vi "Main.vi"() -> ()   [LabVIEW 2015]
doc: "The myRIO Project template acquires acceleration data from the onboard accelerometer and displays the changes of acceleration values in a waveform chart."
uses:
  <vilib>/myRIO/Instrument Drivers/Onboard IO/PWM/typedefs/PWM Reference.ctl
  <vilib>/myRIO/Common/Instrument Driver Framework/Utilities/typedefs/myRIO Generic Hardware Reference.ctl
  <vilib>/myRIO/Common/Instrument Driver Framework/Utilities/typedefs/Hardware Version Enum.ctl
  <vilib>/myRIO/Common/Instrument Driver Framework/Utilities/typedefs/myRIO v1.0 Reference.ctl
  <vilib>/myRIO/Common/Instrument Driver Framework/Utilities/typedefs/Generic FPGA Reference.ctl
  <vilib>/myRIO/Common/Instrument Driver Framework/myRIO v1.0/PWM/typedefs/PWM Channels Enum.ctl
  <vilib>/myRIO/Instrument Drivers/Onboard IO/PWM/typedefs/PWM Configuration.ctl
  <vilib>/userdefined/High Color/nirio_resource_hc.ctl
  <vilib>/myRIO/Instrument Drivers/Onboard IO/AI/typedefs/AI Reference.ctl
  <vilib>/myRIO/Common/Instrument Driver Framework/myRIO v1.0/AI/typedefs/AI Channels List.ctl
  <vilib>/myRIO/Common/Instrument Driver Framework/myRIO v1.0/AI/typedefs/AI Channels Enum.ctl
  <vilib>/myRIO/Common/Instrument Driver Framework/Utilities/typedefs/Analog Scaling Constants List.ctl
  <vilib>/myRIO/Common/Instrument Driver Framework/Utilities/typedefs/Analog Scaling Constants.ctl
  <vilib>/myRIO/Instrument Drivers/Onboard IO/DIO/typedefs/DIO Reference.ctl
  <vilib>/myRIO/Common/Instrument Driver Framework/myRIO v1.0/DIO/typedefs/DIO Channels List.ctl
  <vilib>/myRIO/Common/Instrument Driver Framework/myRIO v1.0/DIO/typedefs/DIO Channels Enum.ctl
  <vilib>/myRIO/Instrument Drivers/Onboard Devices/Accelerometer/typedefs/Accelerometer Reference.ctl
  <vilib>/myRIO/Common/Instrument Driver Framework/myRIO v1.0/Accelerometer/typedefs/Accelerometer Channels List.ctl
  <vilib>/myRIO/Common/Instrument Driver Framework/myRIO v1.0/Accelerometer/typedefs/Accelerometer Channels Enum.ctl
  <vilib>/myRIO/Common/Instrument Driver Framework/Utilities/vis/Is FPGA Ref Available.vi
  <vilib>/myRIO/Common/Instrument Driver Framework/myRIO v1.0/DIO/vis/myRIO v1.1 Open DIO.vi
  <vilib>/myRIO/Instrument Drivers/Onboard IO/DIO/vis/Write.vi
  <vilib>/myRIO/Instrument Drivers/Onboard IO/DIO/vis/Read.vi
  <vilib>/myRIO/Common/Instrument Driver Framework/myRIO v1.0/PWM/vis/myRIO v1.1 Open PWM.vi
  <vilib>/myRIO/Instrument Drivers/Onboard IO/PWM/vis/Set Duty Cycle and Frequency.vi
  <vilib>/myRIO/Common/Instrument Driver Framework/myRIO v1.0/AI/vis/myRIO v1.1 Open AI.vi
  <vilib>/myRIO/Instrument Drivers/Onboard IO/AI/vis/Read.vi
  <vilib>/myRIO/Common/Instrument Driver Framework/myRIO v1.0/Accelerometer/vis/myRIO v1.1 Open Accelerometer.vi
  <vilib>/myRIO/Instrument Drivers/Onboard Devices/Accelerometer/vis/Read.vi
  <vilib>/myRIO/Common/Instrument Driver Framework/Utilities/vis/Validate Channels.vi
  <vilib>/myRIO/Common/Instrument Driver Framework/myRIO v1.0/DIO/vis/myRIO v1.0 Reserve DIO.vi
  <vilib>/myRIO/Common/Instrument Driver Framework/myRIO v1.0/PWM/vis/myRIO v1.0 Reserve PWM.vi
  <vilib>/myRIO/Common/Instrument Driver Framework/myRIO v1.0/AI/vis/myRIO v1.0 Reserve AI.vi
  <vilib>/myRIO/Common/Instrument Driver Framework/myRIO v1.0/Accelerometer/vis/myRIO v1.0 Reserve Accelerometer.vi
  <vilib>/myRIO/Common/Instrument Driver Framework/myRIO v1.0/UART/vis/myRIO v1.0 Close UART.vi
  <vilib>/myRIO/Common/Instrument Driver Framework/myRIO v1.0/Resource Manager/vis/myRIO v1.0 Reserve Channel List.vi
  <vilib>/myRIO/Common/Instrument Driver Framework/myRIO v1.0/DIO/vis/myRIO v1.0 Build MUX Configuration DIO.vi
  <vilib>/myRIO/Common/Instrument Driver Framework/myRIO v1.0/PWM/vis/myRIO v1.0 Build MUX Configuration PWM.vi
  <vilib>/myRIO/Common/Instrument Driver Framework/myRIO v1.0/AI/vis/myRIO v1.0 Build MUX Configuration AI.vi
  <vilib>/myRIO/Common/Instrument Driver Framework/myRIO v1.0/Accelerometer/vis/myRIO v1.0 Build MUX Configuration Accelerometer.vi
  <vilib>/myRIO/Common/Instrument Driver Framework/myRIO v1.0/Resource Manager/vis/myRIO v1.0 Reserve Channel.vi
  <vilib>/myRIO/Common/Instrument Driver Framework/myRIO v1.0/Resource Manager/vis/myRIO v1.0 Unreserve Channel.vi
  <vilib>/myRIO/Common/Instrument Driver Framework/myRIO v1.0/Resource Manager/vis/myRIO v1.0 Create Configuration List.vi
  <vilib>/myRIO/Common/Instrument Driver Framework/myRIO v1.0/Resource Manager/vis/myRIO v1.0 Build Mutex Name.vi
  <vilib>/Utility/VariantDataType/GetNumericInfo.vi
  <vilib>/Utility/error.llb/Error Cluster From Error Code.vi
  <vilib>/myRIO/Common/Instrument Driver Framework/myRIO v1.0/myRIO v1.1 Open.vi
  <vilib>/myRIO/Common/Instrument Driver Framework/Utilities/vis/IO Manager.vi
  <vilib>/myRIO/Common/Instrument Driver Framework/Utilities/vis/Configuration Manager.vi
  <vilib>/myRIO/Common/Instrument Driver Framework/myRIO v1.0/Resource Manager/vis/myRIO v1.0 Configure IO.vi
  <vilib>/myRIO/Common/Instrument Driver Framework/myRIO v1.0/myRIO v1.0 Close.vi
  <vilib>/myRIO/Common/Instrument Driver Framework/myRIO v1.0/PWM/vis/myRIO v1.0 Write PWM.vi
  <vilib>/myRIO/Common/Instrument Driver Framework/myRIO v1.0/AI/vis/myRIO v1.0 Get Scaling Constants AI.vi
  <vilib>/myRIO/Common/Instrument Driver Framework/myRIO v1.0/AI/vis/myRIO v1.0 Read AI.vi
  <vilib>/addons/control/pid/pid.llb/PID (DBL).vi
  <vilib>/myRIO/Common/Instrument Driver Framework/myRIO v1.0/DIO/vis/myRIO v1.0 Read DIO.vi
  <vilib>/myRIO/Common/Instrument Driver Framework/myRIO v1.0/DIO/vis/myRIO v1.0 Write DIO.vi
  <vilib>/myRIO/Common/Instrument Driver Framework/myRIO v1.0/Accelerometer/vis/myRIO v1.0 Get Scaling Constant Accelerometer.vi
  <vilib>/myRIO/Common/Instrument Driver Framework/myRIO v1.0/Accelerometer/vis/myRIO v1.0 Read Accelerometer.vi
  <vilib>/myRIO/Common/Instrument Driver Framework/Utilities/vis/FPGA Ref Manager.vi
  <vilib>/myRIO/Common/Instrument Driver Framework/myRIO v1.0/myRIO v1.0 Reset FPGA.vi
  <vilib>/myRIO/Common/Instrument Driver Framework/myRIO v1.0/IRQ/vis/myRIO v1.0 IRQ Info FGV.vi
  <vilib>/myRIO/Common/Instrument Driver Framework/myRIO v1.0/IRQ/vis/myRIO v1.0 Timer IRQ Info FGV.vi
  <vilib>/myRIO/Common/Instrument Driver Framework/myRIO v1.0/IRQ/vis/myRIO v1.0 ISR Agent.vi
  <vilib>/myRIO/Express VI/Onboard IO/PWM/PWM Express VI.xnode
  <vilib>/myRIO/Instrument Drivers/Onboard IO/PWM/vis/myRIO PWM Open.xnode
  <vilib>/myRIO/Express VI/Onboard IO/AI/AI Express VI.xnode
  <vilib>/myRIO/Instrument Drivers/Onboard IO/AI/vis/myRIO AI Open.xnode
  <vilib>/myRIO/Express VI/Onboard IO/DI/DI Express VI.xnode
  <vilib>/myRIO/Instrument Drivers/Onboard IO/DIO/vis/myRIO DIO Open.xnode
  <vilib>/myRIO/Express VI/Onboard IO/DO/DO Express VI.xnode
  <vilib>/myRIO/Express VI/Onboard Devices/Accelerometer/Accelerometer Express VI.xnode
  <vilib>/myRIO/Instrument Drivers/Onboard Devices/Accelerometer/vis/myRIO Accelerometer Open.xnode
  <vilib>/myRIO/Instrument Drivers/Utilities/Utilities.lvlib
  <vilib>/myRIO/Instrument Drivers/Onboard Devices/Accelerometer/Accelerometer.lvlib
  <vilib>/myRIO/Instrument Drivers/Onboard IO/PWM/PWM.lvlib
  <vilib>/myRIO/Instrument Drivers/Onboard IO/DIO/DIO.lvlib
  <vilib>/myRIO/Instrument Drivers/Onboard IO/AI/AI.lvlib
  <vilib>/addons/control/pid/NI_PID_pid.lvlib
panel:
  in  "turn":bool
  out "波形图表 2":dbl(graph)
  out "波形图表":dbl(graph)
  out "数值 3":dbl
  out "数值 2":dbl
  out "数值":dbl
  in  "PID gains":T1={"proportional gain (Kc)"=1.0, "integral time (Ti, min)"=0.01, "derivative time (Td, min)"=0.0} caption="PID增益" {"derivative time (Td, min)" format="%.3f"; "integral time (Ti, min)" format="%.3f"; "proportional gain (Kc)" format="%.3f"}
  out "Acceleration":T2(graph)
  out "error out":errorcluster
  in  "Stop":bool
  # "Overview: The myRIO Project template acquires acceleration data from the onboard accelerometer and displays the changes of acceleration values in a waveform chart.\nInstructions:\n1. Check the myRIO target IP address in the project and make sure the target IP address is correct. \n2. Run this VI."
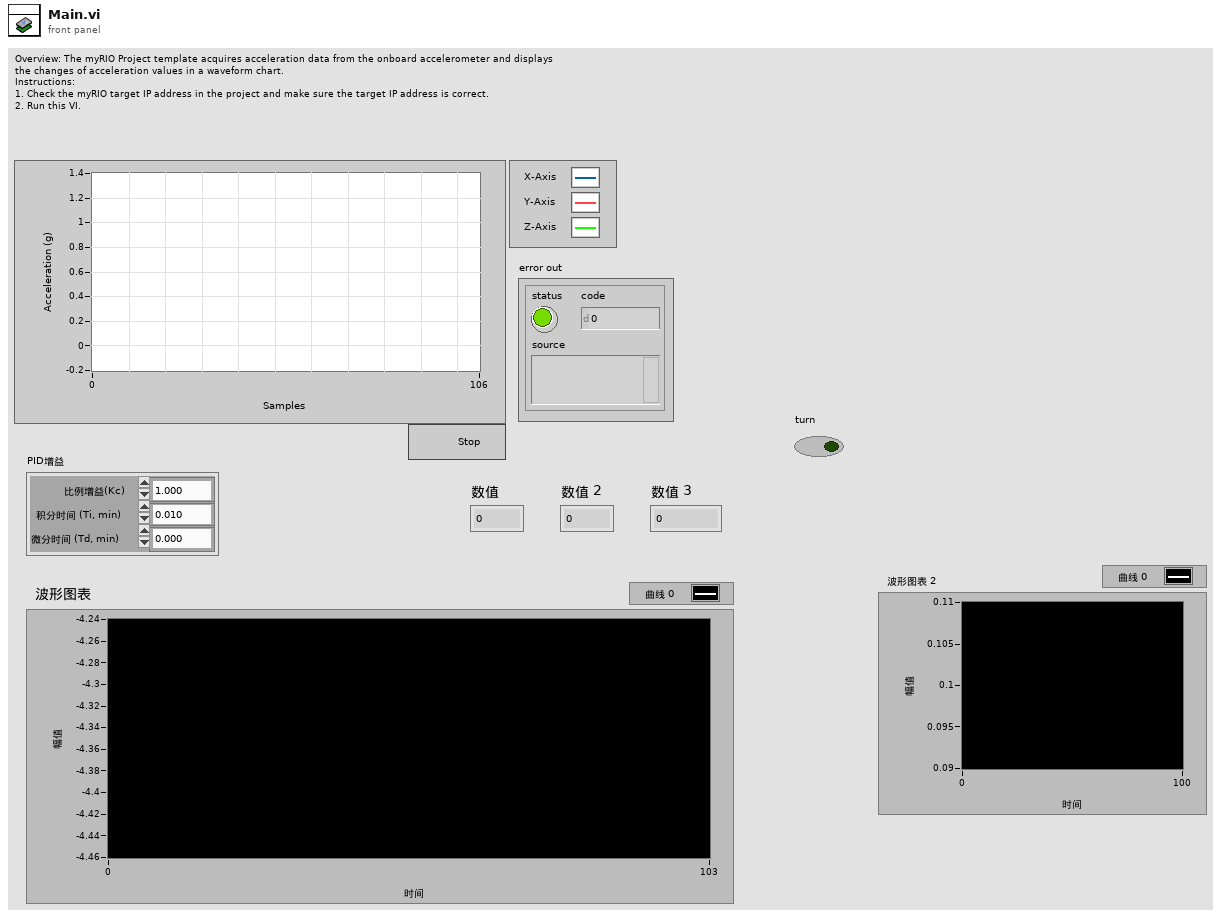
[diagram p1: front panel]
types:
  T1 = cluster{"proportional gain (Kc)":dbl, "integral time (Ti, min)":dbl, "derivative time (Td, min)":dbl}
  T2 = cluster{"X-Axis":dbl, "Y-Axis":dbl, "Z-Axis":dbl}
  T3 = typedef "PWM.lvlib/PWM Reference.ctl" = cluster{"myRIO Reference":T4, "PWM Channels Enum":T8, "PWM Configuration":T9}
  T4 = typedef "myRIO Generic Hardware Reference.ctl" = cluster{"myRIO Model":T5, "myRIO Hardware Reference":T6}
  T5 = typedef "Hardware Version Enum.ctl" = enum16{"Unknown", "myRIO-1900", "myRIO-1950", "roboRIO"}
  T6 = typedef "myRIO v1.0 Reference.ctl" = cluster{"Generic FPGA Reference":T7, "Allow multiple opens":bool}
  T7 = typedef "Generic FPGA Reference.ctl" = refnum<k20>
  T8 = typedef "PWM Channels Enum.ctl" = enum16{"Not Connected", "C/PWM0", "C/PWM1", "A/PWM0", "A/PWM1", "A/PWM2", "B/PWM0", "B/PWM1", "B/PWM2", "PWM/PWM0", "PWM/PWM1", "PWM/PWM2", "PWM/PWM3", "PWM/PWM4", "PWM/PWM5", "PWM/PWM6", "PWM/PWM7", "PWM/PWM8", "PWM/PWM9"}
  T9 = typedef "PWM.lvlib/PWM Configuration.ctl" = cluster{"Frequency":dbl, "Duty Cycle":dbl}
  T10 = typedef "nirio_resource_hc.ctl" = tag
  T11 = typedef "DIO.lvlib/DIO Reference.ctl" = cluster{"myRIO Reference":T4, "DIO Channels List":T12}
  T12 = typedef "DIO Channels List.ctl" = T13[]
  T13 = typedef "DIO Channels Enum.ctl" = enum16{"Not Connected", "C/DIO0", "C/DIO1", "C/DIO2", "C/DIO3", "C/DIO4", "C/DIO5", "C/DIO6", "C/DIO7", "A/DIO0", "A/DIO1", "A/DIO2", "A/DIO3", "A/DIO4", "A/DIO5", "A/DIO6", "A/DIO7", "A/DIO8", "A/DIO9", "A/DIO10", "A/DIO11", "A/DIO12", "A/DIO13", "A/DIO14", "A/DIO15", "B/DIO0", "B/DIO1", "B/DIO2", "B/DIO3", "B/DIO4", "B/DIO5", "B/DIO6", "B/DIO7", "B/DIO8", "B/DIO9", "B/DIO10", "B/DIO11", "B/DIO12", "B/DIO13", "B/DIO14", "B/DIO15", "LED0", "LED1", "LED2", "LED3", "Button0", "DIO/DIO0", "DIO/DIO1", "DIO/DIO2", "DIO/DIO3", "DIO/DIO4", "DIO/DIO5", "DIO/DIO6", "DIO/DIO7", "DIO/DIO8", "DIO/DIO9", "SPI/CS0", "SPI/CS1", "SPI/CS2", "SPI/CS3", "LED RADIO (Green)", "LED RADIO (Red)", "LED COMM (Green)", "LED COMM (Red)", "LED MODE (Green)", "LED MODE (Red)"}
  T14 = typedef "AI.lvlib/AI Reference.ctl" = cluster{"myRIO Reference":T4, "AI Channels List":T15, "AI Scaling Constants List":T17}
  T15 = typedef "AI Channels List.ctl" = T16[]
  T16 = typedef "AI Channels Enum.ctl" = enum16{"Not Connected", "AudioIn/Left", "AudioIn/Right", "C/AI0", "C/AI1", "A/AI0", "A/AI1", "A/AI2", "A/AI3", "B/AI0", "B/AI1", "B/AI2", "B/AI3", "AI/AI0", "AI/AI1", "AI/AI2", "AI/AI3"}
  T17 = typedef "Analog Scaling Constants List.ctl" = T18[]
  T18 = typedef "Analog Scaling Constants.ctl" = cluster{"LSB Weight (Volts)":dbl, "Offset (Volts)":dbl, "Signed?":bool}
  T19 = typedef "Accelerometer.lvlib/Accelerometer Reference.ctl" = cluster{"myRIO Reference":T4, "Accelerometer Channels List":T20, "LSB Weight":dbl}
  T20 = typedef "Accelerometer Channels List.ctl" = T21[]
  T21 = typedef "Accelerometer Channels Enum.ctl" = enum16{"Not Connected", "X-Axis", "Y-Axis", "Z-Axis"}
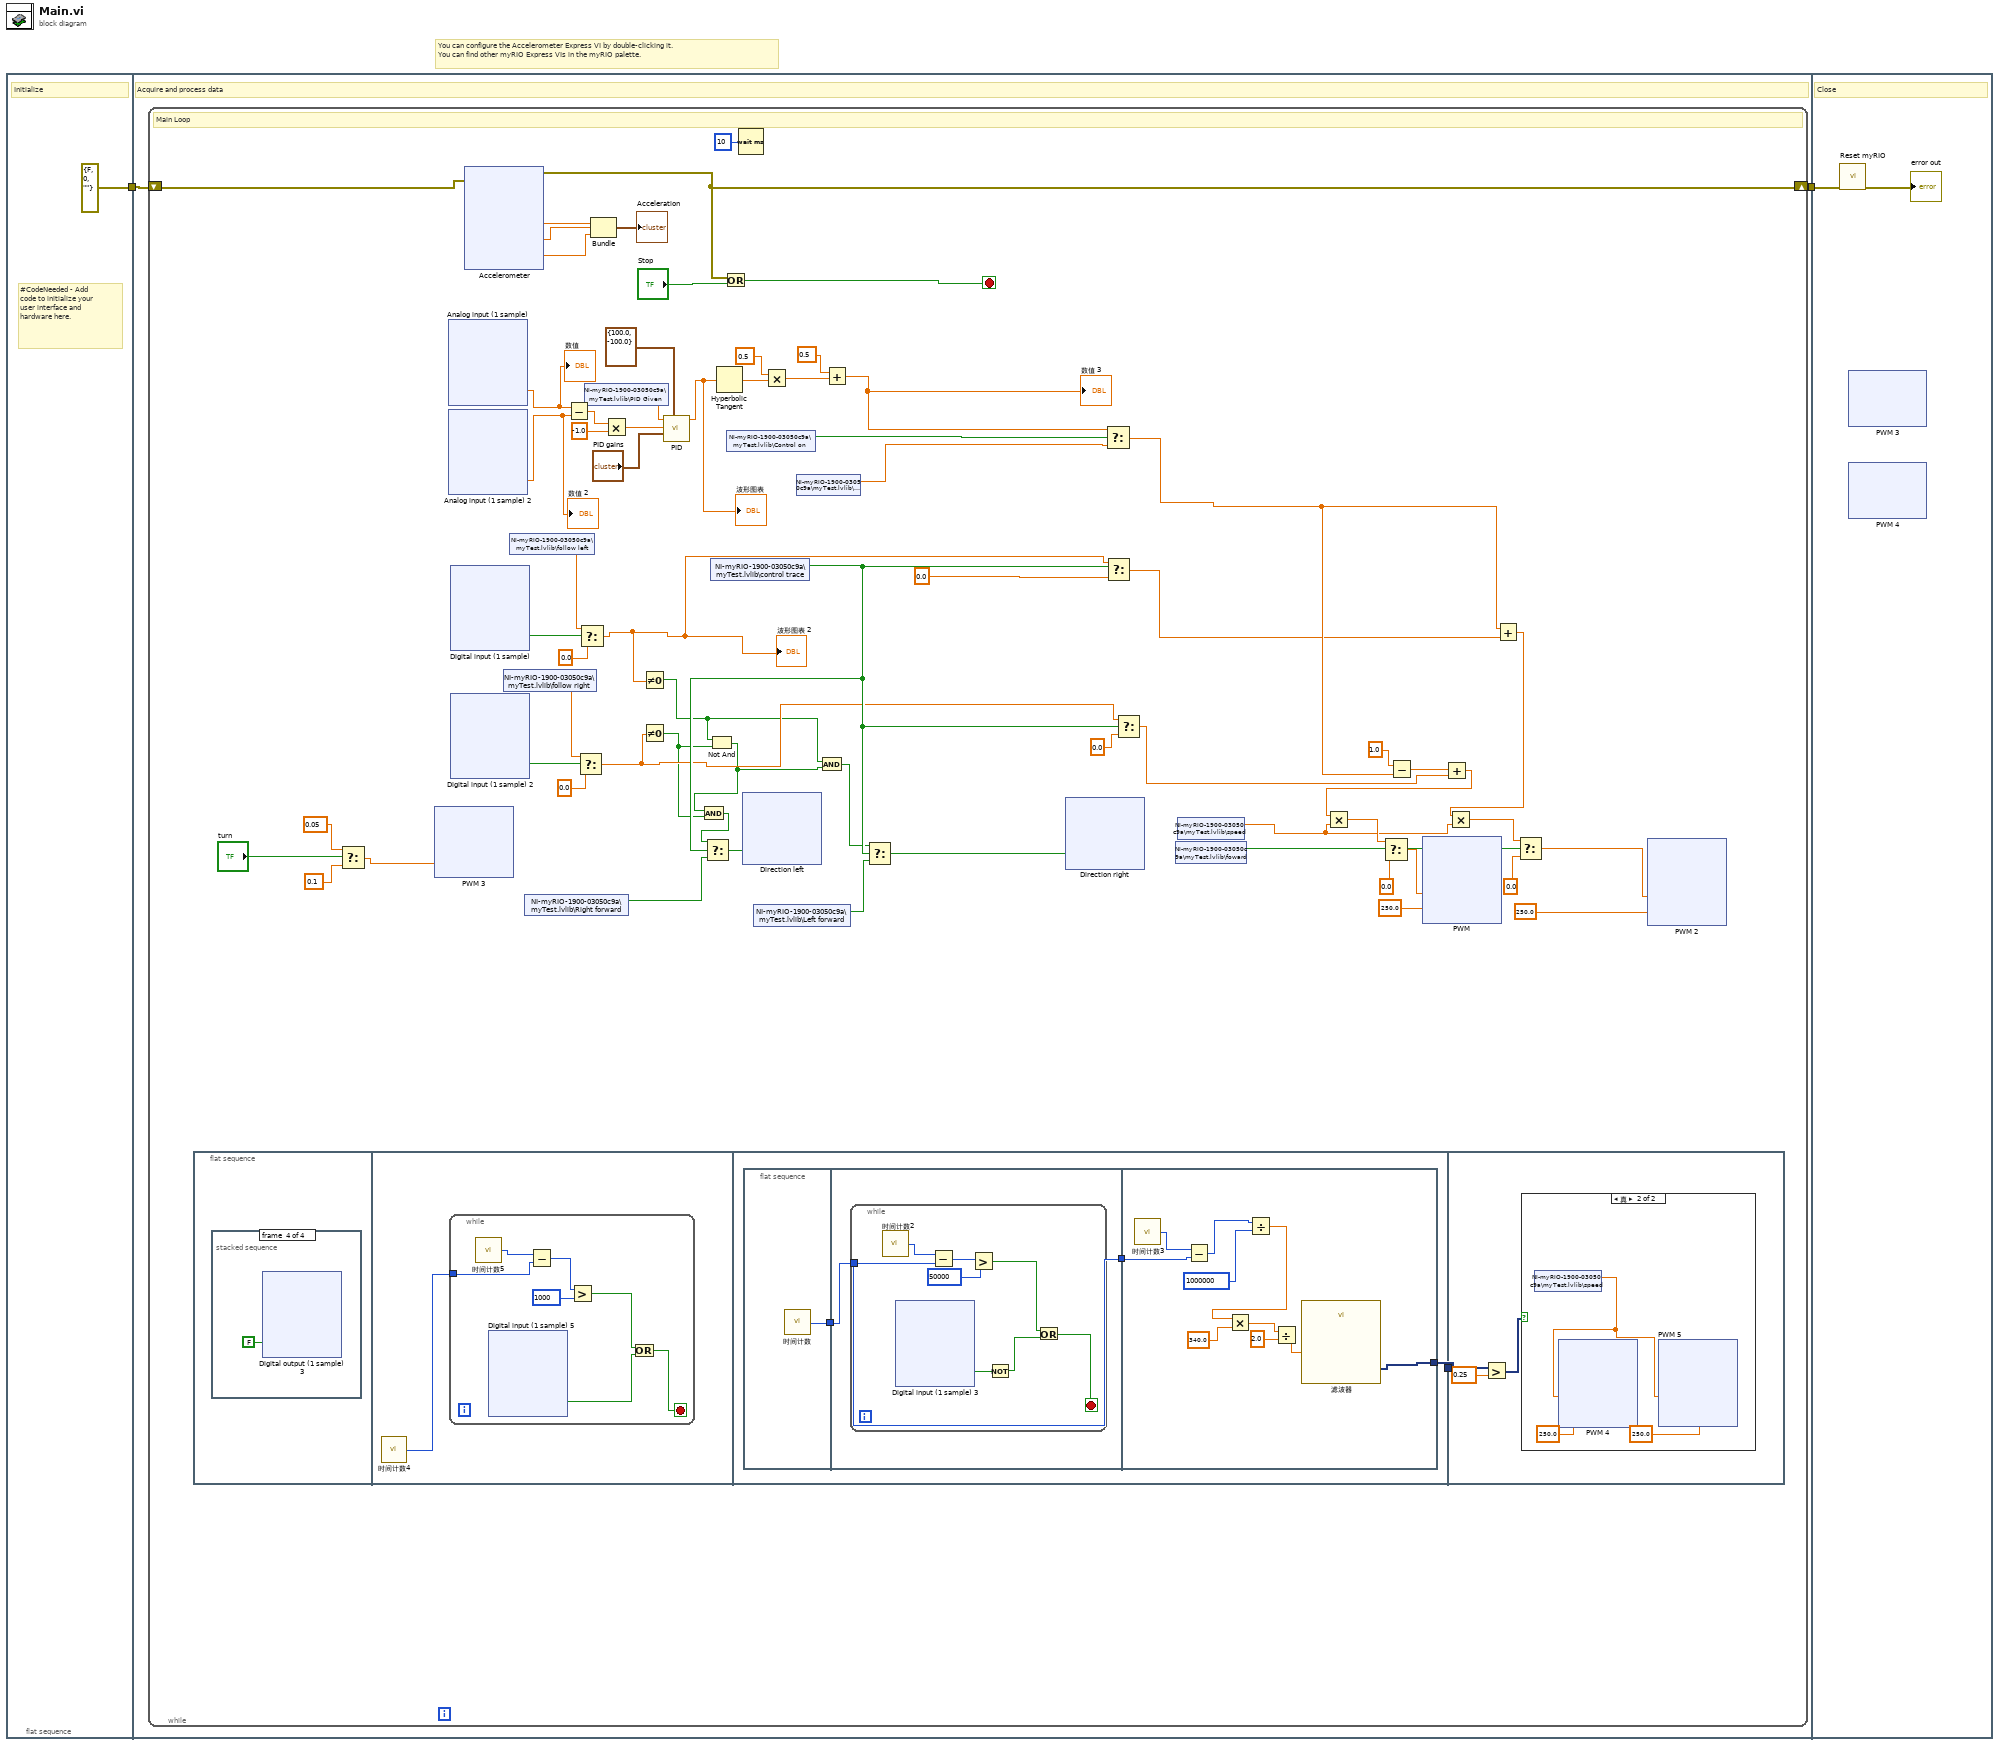
[diagram p0: block diagram]
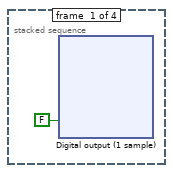
[diagram p2: hidden frame]
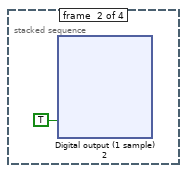
[diagram p3: hidden frame]
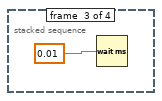
[diagram p4: hidden frame]
diagram:
  # "You can configure the Accelerometer Express VI by double-clicking it.\nYou can find other myRIO Express VIs in the myRIO palette."
  n1 = flat-sequence {
    tunnel: [errorcluster {"status"=FALSE, "code"=0, "source"=""} ("error in (no error)")] -> w2
    tunnel: w2 -> [w5]
    tunnel: [w4] -> w1
    tunnel: w1 -> [w718]
    frame #0 {
      # "#CodeNeeded - Add code to initialize your user interface and hardware here."
      # "Initialize"
    }
    frame #1 {
      # "Acquire and process data"
      n2 = while {
        shift-right: [w68] -> w4
        shift-left: w5 -> [w64]
        stop <- w71 stop-if-true
        # "Main Loop"
        n3 = flat-sequence {
          tunnel: [w260] -> w6
          tunnel: w6 -> [w320]
          frame #0 {
            n4 = stacked-sequence {
              frame #0 {
                n5 = xnode "Digital output (1 sample)"("A/DIO10 (Pin 31)"=FALSE) -> ()  [unwired: 1 in, 1 out]
              }
              frame #1 {
                n6 = xnode "Digital output (1 sample) 2"("A/DIO10 (Pin 31)"=TRUE) -> ()  [unwired: 1 in, 1 out]
              }
              frame #2 {
                n7 = Wait (ms)(milliseconds to wait=0.01 ("等待时间（毫秒）")) -> ()  [unwired: 1 out]
              }
              frame #3 {
                n8 = xnode "Digital output (1 sample) 3"("A/DIO10 (Pin 31)"=FALSE) -> ()  [unwired: 1 in, 1 out]
              }
            }
          }
          frame #1 {
            n9 = call "时间计数4"() -> ("Tick Count(uSec)"=w217:u32)
            n10 = while {
              tunnel: w217 -> [w223]
              stop <- w218 stop-if-true
              n11 = call "时间计数5"() -> ("Tick Count(uSec)"=w224:u32)
              n12 = xnode "Digital input (1 sample) 5"() -> ("A/DIO7 (Pin 25)"=w220:bool)  [unwired: 1 in, 1 out]
              n13 = Subtract(x=w224, y=w223) -> (x-y=w222:u32)
              n14 = Greater?(x=w222, y=u32 1000) -> (0:w219:bool)
              n15 = Or(x=w219, y=w220) -> (x .or. y?=w218:bool)
            }
          }
          frame #2 {
            n16 = flat-sequence {
              tunnel: [w263] -> w262
              tunnel: w262 -> [w264]
              tunnel: [w264] -> w261
              tunnel: w261 -> [w316]
              tunnel: [w308] -> w260
              frame #0 {
                n17 = call "时间计数"() -> ("Tick Count(uSec)"=w263:u32)
              }
              frame #1 {
                n18 = while {
                  tunnel: w264 -> [w271]
                  stop <- w265 stop-if-true
                  n19 = call "时间计数2"() -> ("Tick Count(uSec)"=w272:u32)
                  n20 = xnode "Digital input (1 sample) 3"() -> ("A/DIO7 (Pin 25)"=w268:bool)  [unwired: 1 in, 1 out]
                  n21 = Subtract(x=w272, y=w271) -> (x-y=w270:u32)
                  n22 = Greater?(x=w270, y=u32 50000) -> (0:w267:bool)
                  n23 = Not(x=w268) -> (.not. x?=w266:bool)
                  n24 = Or(x=w267, y=w266) -> (x .or. y?=w265:bool)
                }
              }
              frame #2 {
                n25 = call "时间计数3"() -> ("Tick Count(uSec)"=w317:u32)
                n26 = Subtract(x=w317, y=w316) -> (x-y=w315:u32)
                n27 = Divide(x=w315, y=u32 1000000) -> (x/y=w311:dbl)
                n28 = Multiply(x=w311, y=340.0) -> (x*y=w312:dbl)
                n29 = Divide(x=w312, y=2.0) -> (x/y=w309:dbl)
                n30 = call "滤波器"("Signal"=w309) -> ("Filtered Signal"=w308:dynamicdata)  [unwired: 9 in, 1 out]
              }
            }
          }
          frame #3 {
            n31 = Greater?(x=w320, y=0.25) -> (0:w318:dynamicdata)
            n32 = case shown="真" w318 {
              frame False {
              }
              frame True {
                n33 = shared-variable "NI-myRIO-1900-03050c9a\\myTest.lvlib\\speed"() -> (w321:dbl)  [unwired: 1 in, 1 out]
                n34 = xnode "PWM 4"("Duty Cycle"=w321, "Frequency [Hz]"=250.0) -> ()  [unwired: 1 in, 1 out]
                n35 = xnode "PWM 5"("Duty Cycle"=w321, "Frequency [Hz]"=250.0) -> ()  [unwired: 1 in, 1 out]
              }
            }
          }
        }
        n36 = Select(t=0.05, s="turn", f=0.1) -> (s? t:f=w10:dbl)
        n37 = xnode "PWM 3"("Duty Cycle"=w10) -> ()  [unwired: 1 in, 1 out]
        n38 = xnode "Analog input (1 sample)"() -> ("A/AI2 (Pin 7)"=w47:dbl)  [unwired: 1 in, 1 out]
        "数值" <- w47
        n39 = xnode "Analog input (1 sample) 2"() -> ("A/AI1 (Pin 5)"=w48:dbl)  [unwired: 1 in, 1 out]
        "数值 2" <- w48
        n40 = xnode "Digital input (1 sample)"() -> ("A/DIO1 (Pin 13)"=w27:bool)  [unwired: 1 in, 1 out]
        n41 = xnode "Digital input (1 sample) 2"() -> ("A/DIO0 (Pin 11)"=w28:bool)  [unwired: 1 in, 1 out]
        n42 = xnode "Accelerometer"("error in (no error)"=w64) -> ("X-Axis"=w66:dbl, "Y-Axis"=w65:dbl, "Z-Axis"=w67:dbl, "error out"=w68:errorcluster)
        n43 = shared-variable "NI-myRIO-1900-03050c9a\\myTest.lvlib\\follow right"() -> (w23:dbl)  [unwired: 1 in, 1 out]
        n44 = shared-variable "NI-myRIO-1900-03050c9a\\myTest.lvlib\\follow left"() -> (w24:dbl)  [unwired: 1 in, 1 out]
        n45 = shared-variable "NI-myRIO-1900-03050c9a\\myTest.lvlib\\Right forward"() -> (w22:bool)  [unwired: 1 in, 1 out]
        n46 = Subtract(x=w47, y=w48) -> (x-y=w40:dbl)
        n47 = Select(t=w23, s=w28, f=0.0 ("x")) -> (s? t:f=w17:dbl)
        n48 = Select(t=w24, s=w27, f=0.0 ("x")) -> (s? t:f=w16:dbl)
        "波形图表 2" <- w16
        n49 = shared-variable "NI-myRIO-1900-03050c9a\\myTest.lvlib\\PID Given"() -> (w41:dbl)  [unwired: 1 in, 1 out]
        n50 = Bundle("X-Axis"=w66, "Y-Axis"=w65, "Z-Axis"=w67) -> (→"Acceleration":T2)  [unwired: 1 in]
        n51 = Multiply(x=w40, y=-1.0) -> (x*y=w38:dbl)
        n52 = Not Equal To 0?(x=w16) -> (x != 0?=w13:bool)
        n53 = Not Equal To 0?(x=w17) -> (x != 0?=w15:bool)
        n54 = call-poly <vilib>:"PID.vi"("output range"=cluster{"output high":dbl, "output low":dbl} {"output high"=100.0, "output low"=-100.0}, "PID gains"="PID gains", "process variable"=w38, "setpoint"=w41) -> ("output"=w42:dbl)  [unwired: 6 in, 1 out]
        "波形图表" <- w42
        n55 = Not And(1:w15, 2:w13) -> (0:w12:bool)
        n56 = And(x=w12, y=w15) -> (x .and. y?=w14:bool)
        n57 = shared-variable "NI-myRIO-1900-03050c9a\\myTest.lvlib\\control trace"() -> (w18:bool)  [unwired: 1 in, 1 out]
        n58 = Select(t=w14, s=w18, f=w22) -> (s? t:f=w21:bool)
        n59 = Hyperbolic Tangent(1:w42) -> (0:w45:dbl)
        n60 = Or(x=w68, y="Stop") -> (x .or. y?=w71:bool)
        n61 = shared-variable "NI-myRIO-1900-03050c9a\\myTest.lvlib\\Control on"() -> (w50:bool)  [unwired: 1 in, 1 out]
        n62 = Wait (ms)(milliseconds to wait=u32 10) -> ()  [unwired: 1 out]
        n63 = xnode "Direction left"("B/DIO3 (Pin 17)"=w21) -> ()  [unwired: 1 in, 1 out]
        n64 = shared-variable "NI-myRIO-1900-03050c9a\\myTest.lvlib\\Left forward"() -> (w19:bool)  [unwired: 1 in, 1 out]
        n65 = Multiply(x=0.5, y=w45) -> (x*y=w43:dbl)
        n66 = shared-variable "NI-myRIO-1900-03050c9a\\myTest.lvlib\\angle"() -> (w49:dbl)  [unwired: 1 in, 1 out]
        n67 = And(x=w13, y=w12) -> (x .and. y?=w11:bool)
        n68 = Add(x=0.5, y=w43) -> (x+y=w46:dbl)
        "数值 3" <- w46
        n69 = Select(t=w11, s=w18, f=w19) -> (s? t:f=w20:bool)
        n70 = xnode "Direction right"("A/DIO3 (Pin 17)"=w20) -> ()  [unwired: 1 in, 1 out]
        n71 = Select(t=w46, s=w50, f=w49) -> (s? t:f=w31:dbl)
        n72 = Select(t=w16, s=w18, f=0.0) -> (s? t:f=w30:dbl)
        n73 = Select(t=w17, s=w18, f=0.0) -> (s? t:f=w29:dbl)
        n74 = shared-variable "NI-myRIO-1900-03050c9a\\myTest.lvlib\\foward"() -> (w57:bool)  [unwired: 1 in, 1 out]
        n75 = shared-variable "NI-myRIO-1900-03050c9a\\myTest.lvlib\\speed"() -> (w37:dbl)  [unwired: 1 in, 1 out]
        n76 = Subtract(x=1.0, y=w31) -> (x-y=w33:dbl)
        n77 = Add(x=w33, y=w29) -> (x+y=w32:dbl)
        n78 = Multiply(x=w32, y=w37) -> (x*y=w55:dbl)
        n79 = Select(t=w55, s=w57, f=0.0) -> (s? t:f=w58:dbl)
        n80 = xnode "PWM"("Duty Cycle"=w58, "Frequency [Hz]"=250.0) -> ()  [unwired: 1 in, 1 out]
        n81 = Add(x=w31, y=w30) -> (x+y=w34:dbl)
        n82 = Multiply(x=w34, y=w37) -> (x*y=w54:dbl)
        n83 = Select(t=w54, s=w57, f=0.0) -> (s? t:f=w59:dbl)
        n84 = xnode "PWM 2"("Duty Cycle"=w59, "Frequency [Hz]"=250.0) -> ()  [unwired: 1 in, 1 out]
      }
    }
    frame #2 {
      # "Close"
      n85 = call <vilib>:"Reset myRIO.vi"("error in (no error)"=w718) -> ("error out"=→"error out":errorcluster)  [unwired: 10 in]
      n86 = xnode "PWM 3"() -> ()  [unwired: 1 in, 1 out]
      n87 = xnode "PWM 4"() -> ()  [unwired: 1 in, 1 out]
    }
  }
